vi "Function Waveform Generator VI.vi"() -> ()   [LabVIEW 2016]
panel:
  out "返回数":u32
  out "读取缓冲区":string
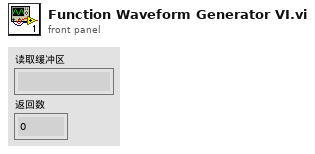
[diagram p1: front panel]
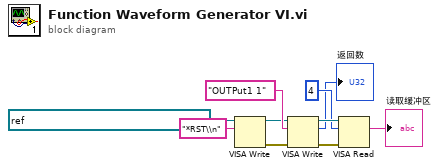
[diagram p0: block diagram]
diagram:
  n1 = VISA Write(VISA resource name=refnum<visa-resource-name> "TCPIP0::192.168.40.227::INSTR" ("VISA资源名称"), write buffer="*RST\\n" ("写入缓冲区")) -> (VISA resource name out=w1:refnum<visa-resource-name>, error out=w3:errorcluster)  [unwired: 1 in, 1 out]
  n2 = VISA Write(VISA resource name=w1, write buffer="OUTPut1 1" ("写入缓冲区"), error in (no error)=w3) -> (VISA resource name out=w9:refnum<visa-resource-name>, return count=→"返回数":u32, error out=w8:errorcluster)
  n3 = VISA Read(VISA resource name=w9, byte count=u32 4 ("字节总数"), error in (no error)=w8) -> (read buffer=→"读取缓冲区":string)  [unwired: 3 out]
